vi "Set Save Settings.vi"(7 "Remove block diagram (true)":bool=TRUE, 8 "error in (no error)":errorcluster, 9 "Remove front panel (true)":bool=TRUE, 10 "ProjectItem Refnum":refnum<vi>, 11 "NI_AB_API_Build in":refnum<class "NI_AB_API_Build.lvclass">) -> (0 "error out":errorcluster, 3 "NI_AB_API_Build out":refnum<class "NI_AB_API_Build.lvclass">)   [LabVIEW 2020, in "NI_AB_API_Build.lvclass"]
uses:
  <vilib>/AppBuilder/AB_API/Build/NI_AB_API_Build.lvclass
  <vilib>/AppBuilder/AB_API/Build/NI_AB_API_Build.lvclass/NI_AB_API_Build.ctl
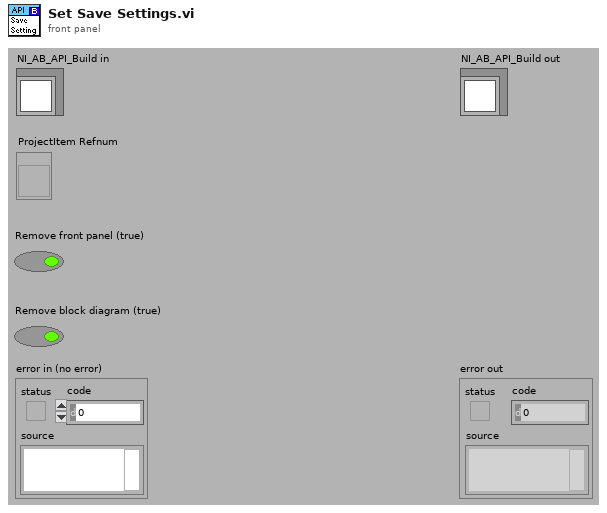
[diagram p1: front panel]
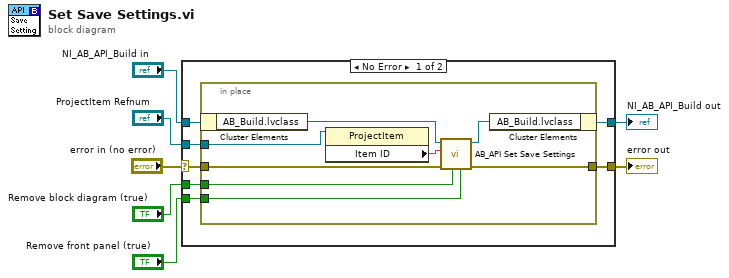
[diagram p0: block diagram]
diagram:
  n1 = case shown="No Error" "error in (no error)" {
    selector: "error in (no error)" -> [w13 w24]
    tunnel: [w14 w24] -> w6
    tunnel: [w8 w23] -> w4
    tunnel: "NI_AB_API_Build in" -> [w9 w23]
    tunnel: "ProjectItem Refnum" -> [w12 _]
    tunnel: "Remove block diagram (true)" -> [w11 _]
    tunnel: "Remove front panel (true)" -> [w10 _]
    frame No Error {
      n2 = in-place {
        in-place-border: [w22] -> w14
        in-place-border: w13 -> [w21]
        in-place-border: w12 -> [w20]
        in-place-border: w11 -> [w19]
        in-place-border: w10 -> [w18]
        n3 = in-place-cluster #1(w9) -> ("AB_Build.lvclass"=w16:refnum<class "AB_Build.lvclass">)
        n4 = property class="ProjectItem"(reference=w20) -> ("Item ID"=w17:string)  [unwired: 1 in, 2 out]
        n5 = call <vilib>:"AB_API Set Save Settings.vi"("Remove front panel (false)"=w18, "Remove block diagram (false)"=w19, "error in (no error)"=w21, "source item ID"=w17, "Build in"=w16) -> ("error out"=w22:errorcluster, "Build out"=w15:refnum<class "AB_Build.lvclass">)  [unwired: 2 in, 3 out]
        n6 = in-place-cluster #1("AB_Build.lvclass"=w15) -> (w8:refnum<class "NI_AB_API_Build.lvclass">)
      }
    }
    frame Error {
    }
  }
  "error out" <- w6
  "NI_AB_API_Build out" <- w4
